vi "ReadWebService.vi"() -> ()   [LabVIEW 2021]
uses:
  <vilib>/httpClient/LabVIEWHTTPClient.lvlib
panel:
  out "Array 2":string[](array[string])
  out "Array":dbl[](array[numeric])
  out "headers":string
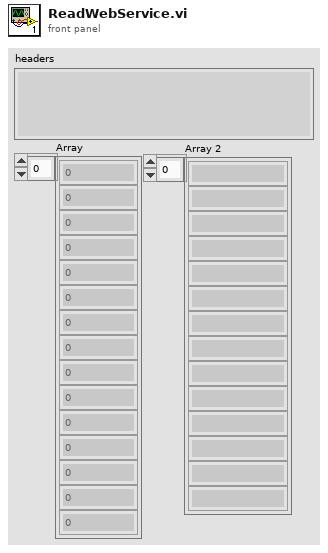
[diagram p1: front panel]
types:
  T1 = typedef "LabVIEWHTTPClient.lvlib/ClientHandle.ctl" = refnum<k1>
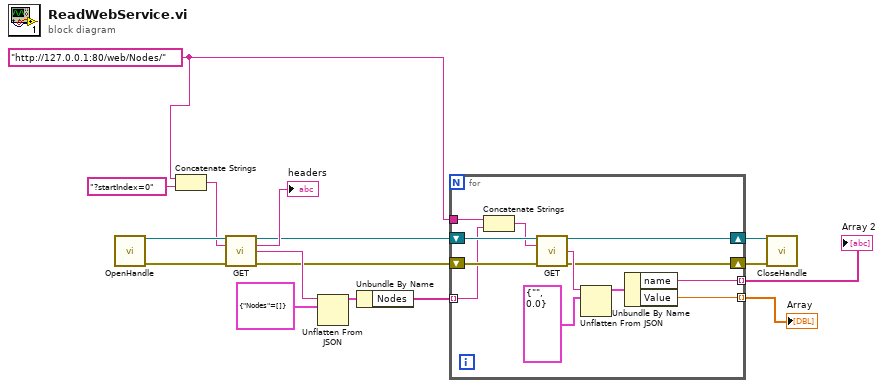
[diagram p0: block diagram]
diagram:
  w1 = "http://127.0.0.1:80/web/Nodes/" ("url")
  n1 = call <vilib>:"OpenHandle.vi"() -> ("client handle out"=w16:T1, "error out"=w15:errorcluster)  [unwired: 14 in]
  n2 = Concatenate Strings(w1, "?startIndex=0" ("string")) -> (w2:string)
  n3 = call <vilib>:"GET.vi"("client handle"=w16, "url"=w2, "error in (no error)"=w15) -> ("client handle out"=w5:T1, "headers"=→"headers":string, "body"=w13:string, "error out"=w6:errorcluster)  [unwired: 9 in]
  n4 = Unflatten From JSON(JSON string=w13, type and defaults=cluster{"Nodes":string[]} {"Nodes"=[]}) -> (value=w9:cluster{"Nodes":string[]})  [unwired: 5 in, 1 out]
  n5 = Unbundle By Name(w9) -> ("Nodes"=w8:string[])
  n6 = for {
    tunnel: w1 -> [w26]
    shift-right: [w19] -> w11
    shift-left: w5 -> [w28]
    shift-right: [w20] -> w10
    shift-left: w6 -> [w27]
    tunnel: w8 -> [w18] mode=indexing
    tunnel: [w21] -> w7 mode=indexing
    tunnel: [w17] -> w4 mode=indexing
    n7 = Concatenate Strings(w26, w18) -> (w25:string)
    n8 = call <vilib>:"GET.vi"("client handle"=w28, "url"=w25, "error in (no error)"=w27) -> ("client handle out"=w19:T1, "body"=w24:string, "error out"=w20:errorcluster)  [unwired: 9 in, 1 out]
    n9 = Unflatten From JSON(JSON string=w24, type and defaults=cluster{"name":string, "Value":dbl} {"name"="", "Value"=0.0}) -> (value=w22:cluster{"name":string, "Value":dbl})  [unwired: 5 in, 1 out]
    n10 = Unbundle By Name(w22) -> ("name"=w17:string, "Value"=w21:dbl)
  }
  "Array" <- w7
  "Array 2" <- w4
  n11 = call <vilib>:"CloseHandle.vi"("client handle"=w11, "error in (no error)"=w10) -> ()  [unwired: 13 in, 1 out]
